vi "Close TDMS.vi"(8 "error in (no error)":errorcluster, 11 "Parallax PING))) in":refnum<class "Parallax PING))).lvclass">) -> (0 "error out":errorcluster, 3 "Parallax PING))) out":refnum<class "Parallax PING))).lvclass">)   [LabVIEW 2013, in "Parallax PING))).lvclass"]
doc: "Closes the tdms file."
uses:
  Parallax PING))).lvclass
  Parallax PING))).lvclass/Parallax PING))).ctl
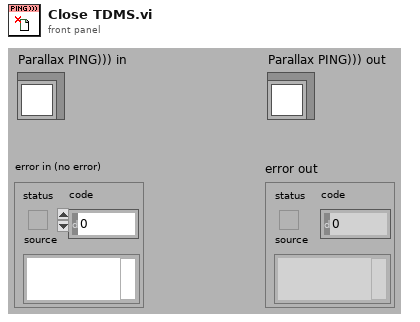
[diagram p1: front panel]
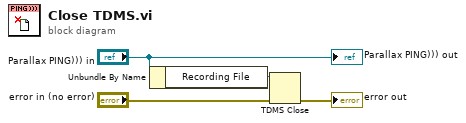
[diagram p0: block diagram]
diagram:
  n1 = Unbundle By Name("Parallax PING))) in") -> ("Recording File"=w1:refnum<k34>)
  n2 = TDMS Close(8:"error in (no error)", 11:w1) -> (0:→"error out":errorcluster)  [unwired: 1 out]
  "Parallax PING))) out" <- "Parallax PING))) in"
